vi "Test Get Failed Items within Library.vi"(11 "Result Model Result Recording Test in":refnum<class "Result Model Result Recording Test.lvclass">) -> (0 "error out":errorcluster, 3 "Result Model Result Recording Test out":refnum<class "Result Model Result Recording Test.lvclass">)   [LabVIEW 2020, in "Result Model Result Recording Test.lvclass"]
uses:
  Result Model Result Recording Test.lvclass
  C:/Program Files (x86)/National Instruments/LabVIEW 2020/vi.lib/Astemes/LUnit/Test Case.lvclass
  source/User Interface/Result Model/Tree Item Filter.ctl
  <vilib>/Astemes/LUnit/Test Case.lvclass/Test Case.ctl
  ae2c71b8-32bb-49d1-8500-0119bfec74ff.vi
  <vilib>/Astemes/LUnit/Core/LUnit Test Case/Private/Append Pass Result.vi
  <vilib>/Astemes/LUnit/Core/LUnit Test Case/Private/Append Fail Result.vi
  ae2c71b8-32bb-49d1-8500-0119bfec74ff.vi/9c5d11cd-9439-4240-a1ee-d9baace9c924.vi
  <vilib>/Astemes/LUnit/Core/LUnit Test Case/Private/Run In UI.vi
  <vilib>/Utility/error.llb/Clear Errors.vi
  source/User Interface/Result Model by Reference/Result Model by Reference.lvclass
  Result Model Result Recording Test.lvclass/Result Model Result Recording Test.ctl
  source/User Interface/Result Model/Result Model.lvclass
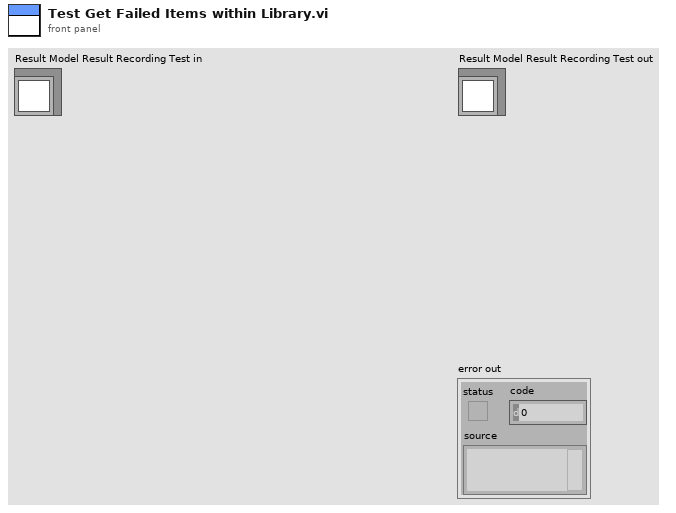
[diagram p1: front panel]
types:
  T1 = cluster{"Name":string, "Description":string, "Status":enum16{"", "Passed", "Failed", "Error", "Skipped", "Setup Error", "Broken", "Teardown Error"}, "Result Type":enum16{"Test Case", "Test Suite", "Test Run", "Pass", "Fail", "Skip", "Pass if", "Fail if", "Pass if Error", "Fail if Error", "Pass if Equal", "Fail if Equal"}, "Execution Time":dbl, "Data":cluster{"Expected":variant, "Actual":variant, "Delta":variant}}[]
  T2 = typedef "Result Model.lvclass/Tree Item Filter.ctl" = enum16{"All", "Only Fails", "Fails or else Not Executed"}
  T3 = cluster{"Left Cell String":string, "Child Text":string[], "Child Tag":string, "Item Indent":i32, "Child Only?":bool, "Glyph Index":i32}[]
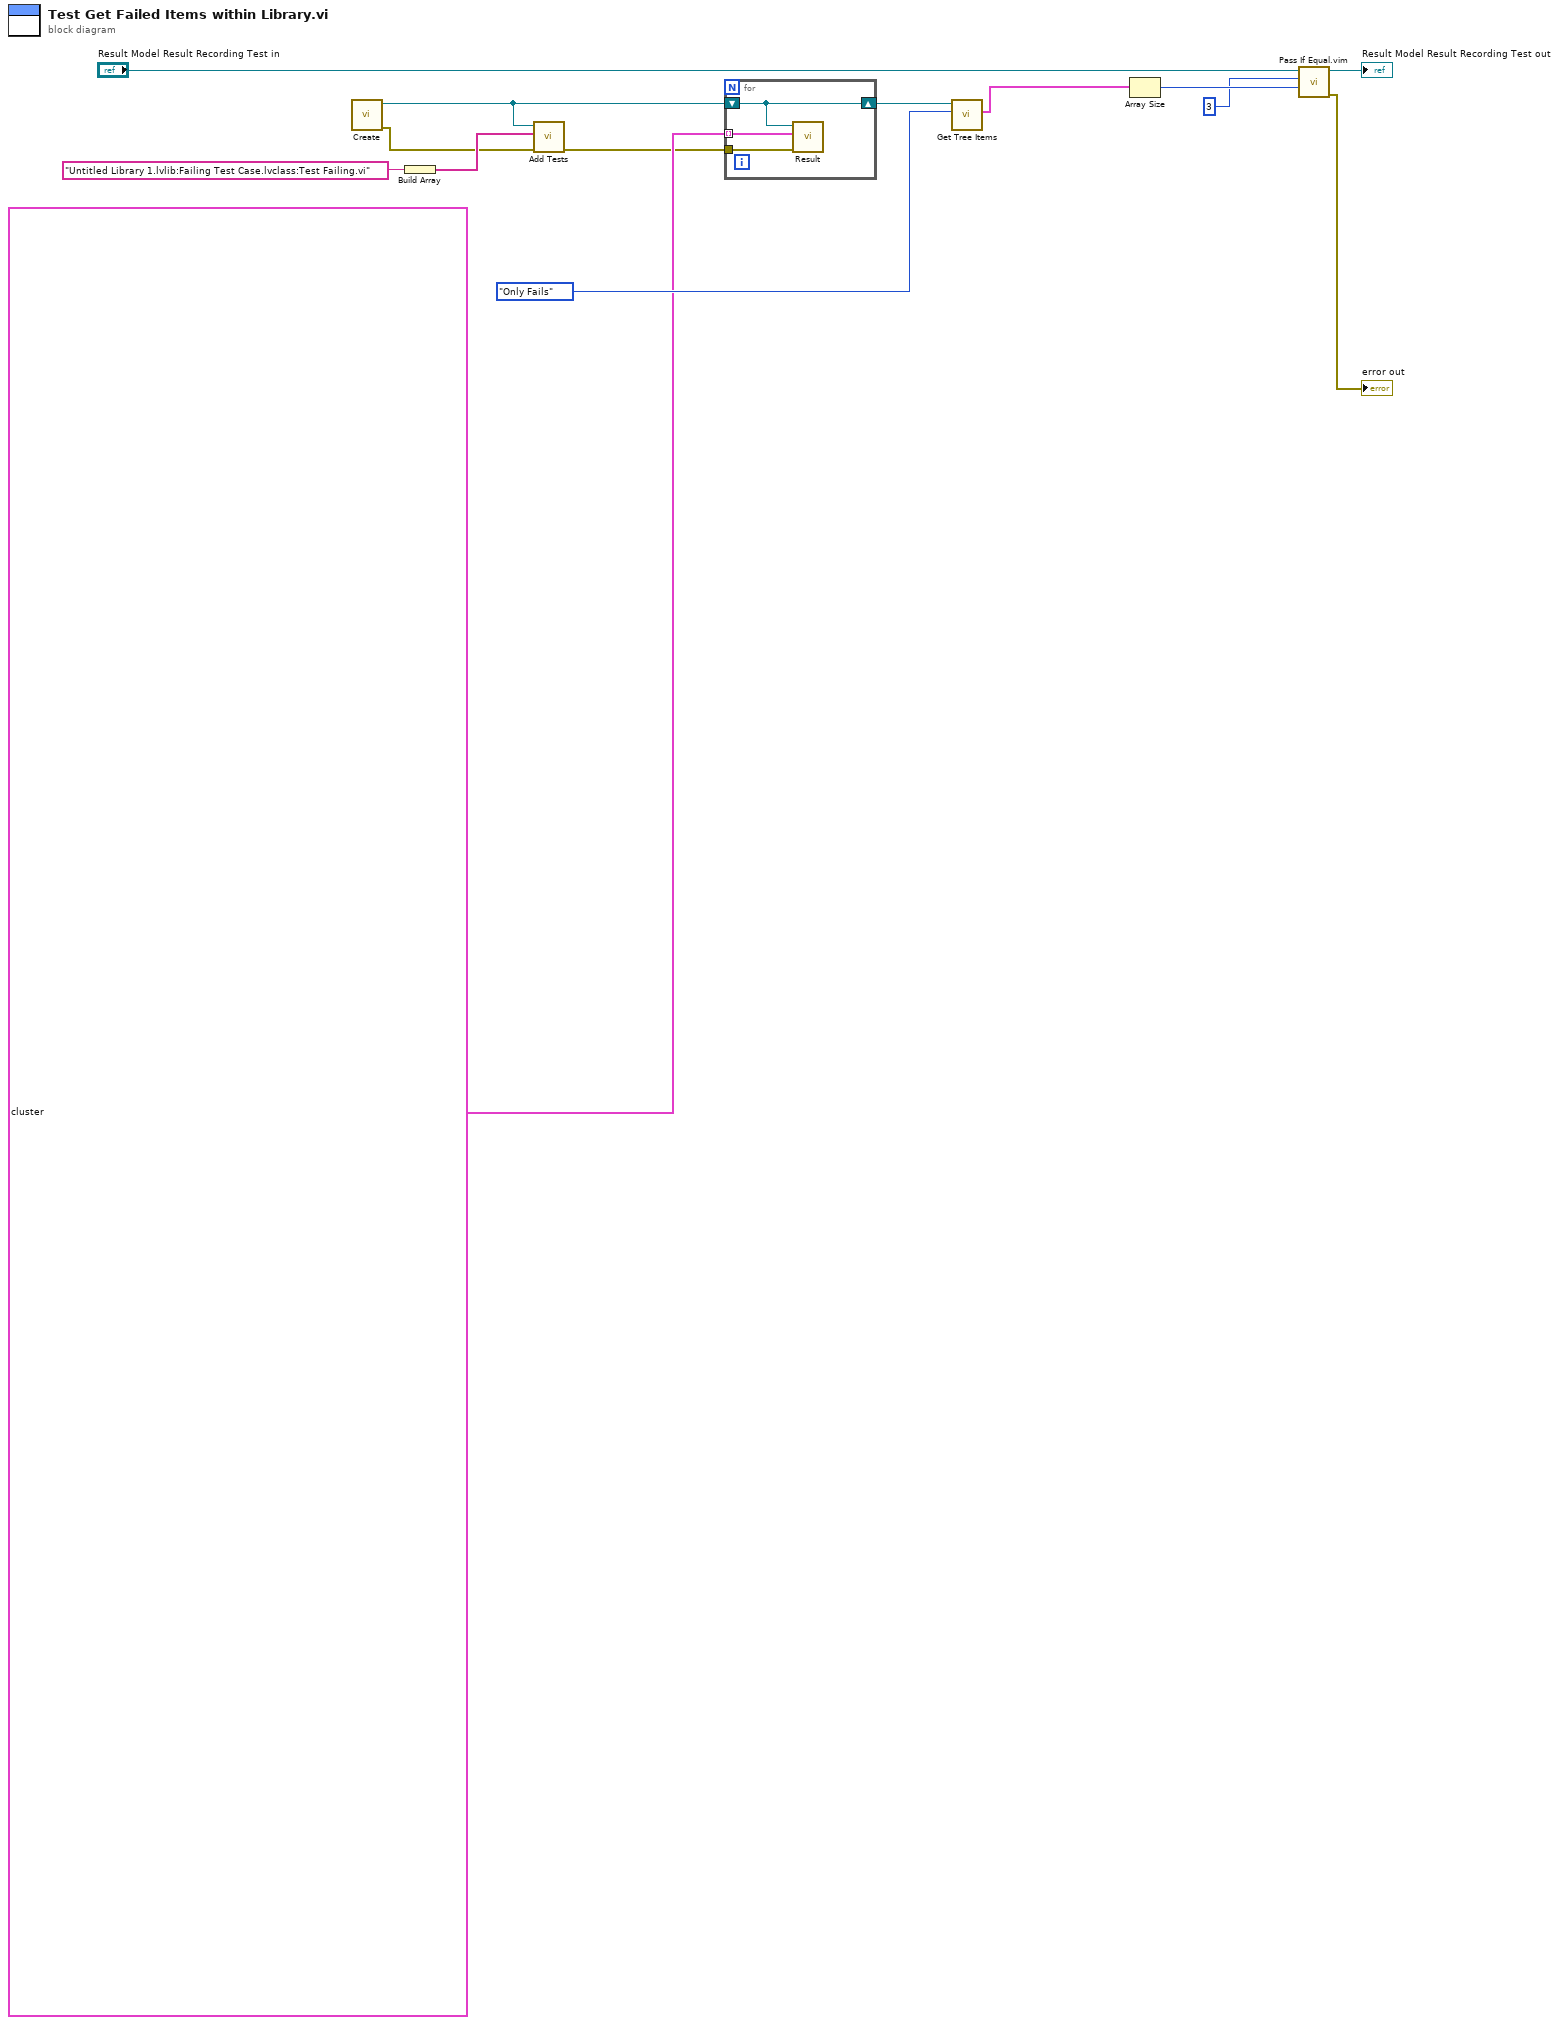
[diagram p0: block diagram]
diagram:
  n1 = call "Create.vi"() -> ("error out"=w1:errorcluster, "Result Model out"=w5:refnum<class "Result Model by Reference.lvclass">)  [unwired: 10 in]
  n2 = Build Array("Untitled Library 1.lvlib:Failing Test Case.lvclass:Test Failing.vi" ("Name")) -> (w3:string[])
  n3 = call "Add Tests.vi"("error in (no error)"=w1, "Tests"=w3, "Result Model by Reference In"=w5) -> ("error out"=w2:errorcluster)  [unwired: 8 in]
  n4 = for {
    tunnel: T1 [{"Name"="Untitled Library 1.lvlib:Failing Test Case.lvclass", "Description"="", "Status"=enum."", "Result Type"=enum."Test Suite", "Execution Time"=0.0, "Data"={"Expected"=variant, "Actual"=variant, "Delta"=variant}}, {"Name"="Untitled Library 1.lvlib:Failing Test Case.lvclass:Test Failing.vi", "Description"="Failing test", "Status"=enum."Failed", "Result Type"=enum."Pass if", "Execution Time"=0.0, "Data"={"Expected"=variant, "Actual"=variant, "Delta"=variant}}, {"Name"="Untitled Library 1.lvlib:Failing Test Case.lvclass:Test Failing.vi", "Description"="Failed:\nFailing test", "Status"=enum."Failed", "Result Type"=enum."Test Case", "Execution Time"=0.009, "Data"={"Expected"=variant, "Actual"=variant, "Delta"=variant}}, {"Name"="Untitled Library 1.lvlib:Failing Test Case.lvclass", "Description"="", "Status"=enum."Failed", "Result Type"=enum."Test Suite", "Execution Time"=0.0, "Data"={"Expected"=variant, "Actual"=variant, "Delta"=variant}}, {"Name"="Untitled Library 1.lvlib:Passing Test Case.lvclass", "Description"="", "Status"=enum."", "Result Type"=enum."Test Suite", "Execution Time"=0.0, "Data"={"Expected"=variant, "Actual"=variant, "Delta"=variant}}, {"Name"="Basic Example.lvproj", "Description"="", "Status"=enum."Failed", "Result Type"=enum."Test Suite", "Execution Time"=0.0, "Data"={"Expected"=variant, "Actual"=variant, "Delta"=variant}}, {"Name"="Untitled Library 1.lvlib:Passing Test Case.lvclass:Test Passing.vi", "Description"="Passing test", "Status"=enum."Passed", "Result Type"=enum."Pass if", "Execution Time"=0.0, "Data"={"Expected"=variant, "Actual"=variant, "Delta"=variant}}, {"Name"="Untitled Library 1.lvlib:Passing Test Case.lvclass:Test Passing.vi", "Description"="Passed:\nPassing test", "Status"=enum."Passed", "Result Type"=enum."Test Case", "Execution Time"=0.008, "Data"={"Expected"=variant, "Actual"=variant, "Delta"=variant}}, {"Name"="Untitled Library 1.lvlib:Passing Test Case.lvclass", "Description"="", "Status"=enum."Passed", "Result Type"=enum."Test Suite", "Execution Time"=0.0, "Data"={"Expected"=variant, "Actual"=variant, "Delta"=variant}}, {"Name"="Untitled Library 1.lvlib", "Description"="", "Status"=enum."Failed", "Result Type"=enum."Test Suite", "Execution Time"=0.0, "Data"={"Expected"=variant, "Actual"=variant, "Delta"=variant}}, {"Name"="Basic Example.lvproj", "Description"="", "Status"=enum."Passed", "Result Type"=enum."Test Suite", "Execution Time"=0.0, "Data"={"Expected"=variant, "Actual"=variant, "Delta"=variant}}] ("appended array") -> [w17] mode=indexing
    shift-right: [w16] -> w14
    shift-left: w5 -> [w16]
    tunnel: w2 -> [w15]
    n5 = call-dynamic "Result.vi"("error in (no error)"=w15, "Results"=w17, "Result Model by Reference In"=w16) -> ()  [unwired: 8 in, 1 out]
  }
  n6 = call "Get Tree Items.vi"("Filter"=Tree_Item_Filter."Only Fails", "Result Model by Reference In"=w14) -> ("Tree Items"=w13:T3)  [unwired: 8 in, 1 out]
  n7 = Array Size(array=w13) -> (size(s)=w9:i32)
  n8 = call "Pass If Equal.vim"("Actual"=w9, "Expected"=3 ("size(s)"), "LUnit Test Case In"="Result Model Result Recording Test in") -> ("error out"=→"error out":errorcluster, "LUnit Test Case Out"=→"Result Model Result Recording Test out":refnum<class "Result Model Result Recording Test.lvclass">)  [unwired: 7 in]
